vi "TestStand_Control ( Load_Seq_File ).vi"(8 "error in (no error)":errorcluster, 10 "sequenceFilePath":string, 11 "TestStand UI Data":T1) -> (0 "error out":errorcluster)   [LabVIEW 2018, in "TestStand_Control.lvlib"]
uses:
  TestStand_Control.lvlib
  Module_Controls/TestStand UI Data.ctl
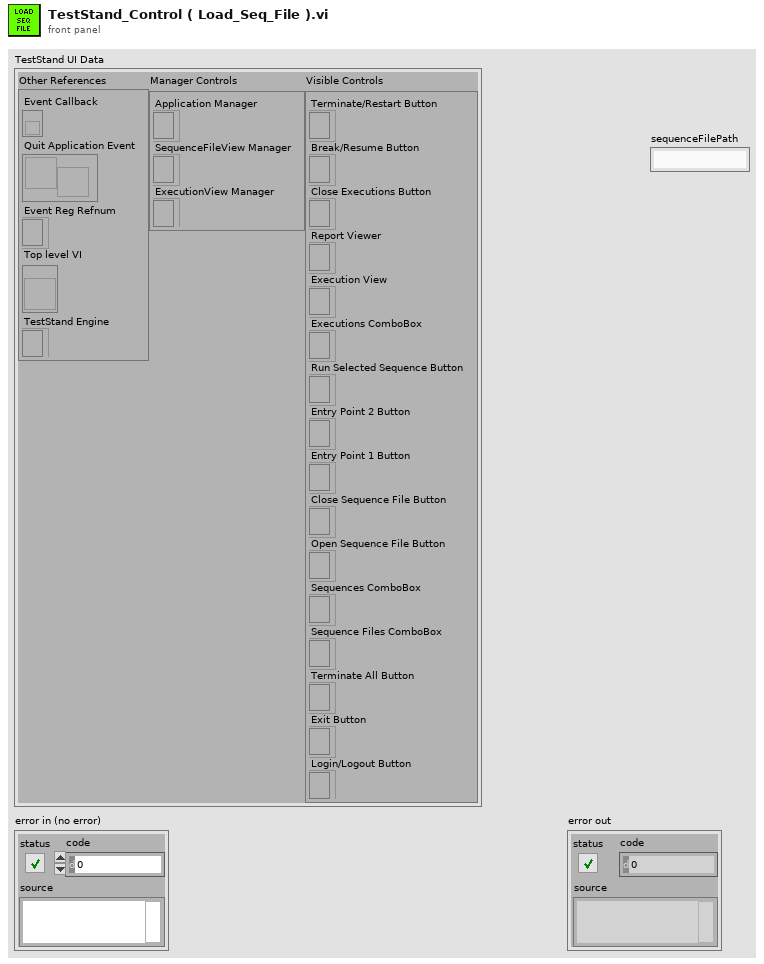
[diagram p1: front panel]
types:
  T1 = typedef "TestStand_Control.lvlib/TestStand UI Data.ctl" = cluster{"Other References":cluster{"Event Callback":refnum<k27>, "Quit Application Event":refnum<user-event>, "Event Reg Refnum":refnum<event-registration>, "Top level VI":refnum<vi>, "TestStand Engine":refnum<k7>}, "Manager Controls":cluster{"Application Manager":refnum<k7>, "SequenceFileView Manager":refnum<k7>, "ExecutionView Manager":refnum<k7>}, "Visible Controls":cluster{"Terminate/Restart Button":refnum<k7>, "Break/Resume Button":refnum<k7>, "Close Executions Button":refnum<k7>, "Report Viewer":refnum<k7>, "Execution View":refnum<k7>, "Executions ComboBox":refnum<k7>, "Run Selected Sequence Button":refnum<k7>, "Entry Point 2 Button":refnum<k7>, "Entry Point 1 Button":refnum<k7>, "Close Sequence File Button":refnum<k7>, "Open Sequence File Button":refnum<k7>, "Sequences ComboBox":refnum<k7>, "Sequence Files ComboBox":refnum<k7>, "Terminate All Button":refnum<k7>, "Exit Button":refnum<k7>, "Login/Logout Button":refnum<k7>}}
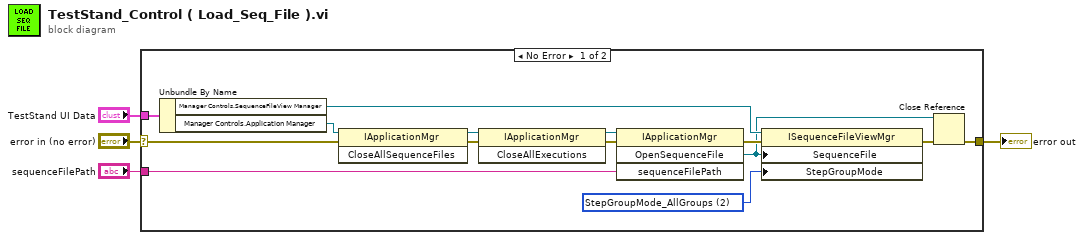
[diagram p0: block diagram]
diagram:
  n1 = case shown="No Error" "error in (no error)" {
    selector: "error in (no error)" -> [w9 w19]
    tunnel: [w8 w19] -> w3
    tunnel: "sequenceFilePath" -> [w7 _]
    tunnel: "TestStand UI Data" -> [w6 _]
    frame No Error {
      w14 = 2 items=["StepGroupMode_OneGroup"=1, "StepGroupMode_AllGroups"=2] ("StepGroupMode")
      n2 = Unbundle By Name(w6) -> ("Manager Controls.SequenceFileView Manager"=w18:refnum<k7>, "Manager Controls.Application Manager"=w5:refnum<k7>)
      n3 = invoke class="IApplicationMgr" method="CloseAllSequenceFiles"(reference=w5, error in=w9) -> (reference out=w12:refnum<k7>, error out=w13:errorcluster)  [unwired: 1 in, 1 out]
      n4 = invoke class="IApplicationMgr" method="CloseAllExecutions"(reference=w12, error in=w13) -> (reference out=w10:refnum<k7>, error out=w11:errorcluster)  [unwired: 1 in, 1 out]
      n5 = invoke class="IApplicationMgr" method="OpenSequenceFile"(reference=w10, error in=w11, "sequenceFilePath"=w7) -> (error out=w16:errorcluster, "OpenSequenceFile"=w15:refnum<k7>)  [unwired: 1 in, 2 out]
      n6 = property class="ISequenceFileViewMgr"(reference=w18, error in=w16, "SequenceFile"=w15, "StepGroupMode"=w14) -> (error out=w17:errorcluster)  [unwired: 1 out]
      n7 = Close Reference(reference=w15, error in (no error)=w17) -> (error out=w8:errorcluster)
    }
    frame Error {
    }
  }
  "error out" <- w3
